vi "main.vi"() -> ()   [LabVIEW 2014]
uses:
  type definitions/control camera properties.ctl
  type definitions/state machine enum.ctl
  <vilib>/userdefined/High Color/IMAQdx.ctl
  <vilib>/vision/driver/NI_Vision_Acquisition_Software.lvlib
panel:
  out "Vertical Pixel Size":dbl
  out "Horizontal Pixel Size":dbl
  out "path":path
  out "bolean intcal":bool
  out "XY Graph":cluster{i32[], u32[]}(graph)
  out "Path to save:":path caption="Path"
  in  "Control Camera Properties":T1={"Packet Size"=1500, "Pixel Format"=17825797, "Gain in dB"=1.0, "Exposure Time in µs"=1500, "Stream Bytes per Second"=50000017} {"Stream Bytes per Second" min=1000000 max=124000000 step=100000 format="%.1p"; "Exposure Time in µs" min=21 max=153391689 format="%#.0f"; "Gain in dB" min=0.0 max=26.0 format="%#_2g"; "Pixel Format" items=["Mono 12 Packed"=17563654, "Mono 12"=17825797]}
  out "Image Pixels (U16)":u16[][](graph)
  in  "Stop Grab 2":bool
  in  "Calibration Button":bool
  out "Camera":T2
  in  "select camera":bool
  in  "Stop Button":bool
  in  "Snap Button":bool
  in  "Grab Button":bool
  in  "Save As Button":bool
  in  "Save Button":bool
  # "Camera Image:"
  # "Spectrum:"
  # "Bytes"
  # "px"
  # "px"
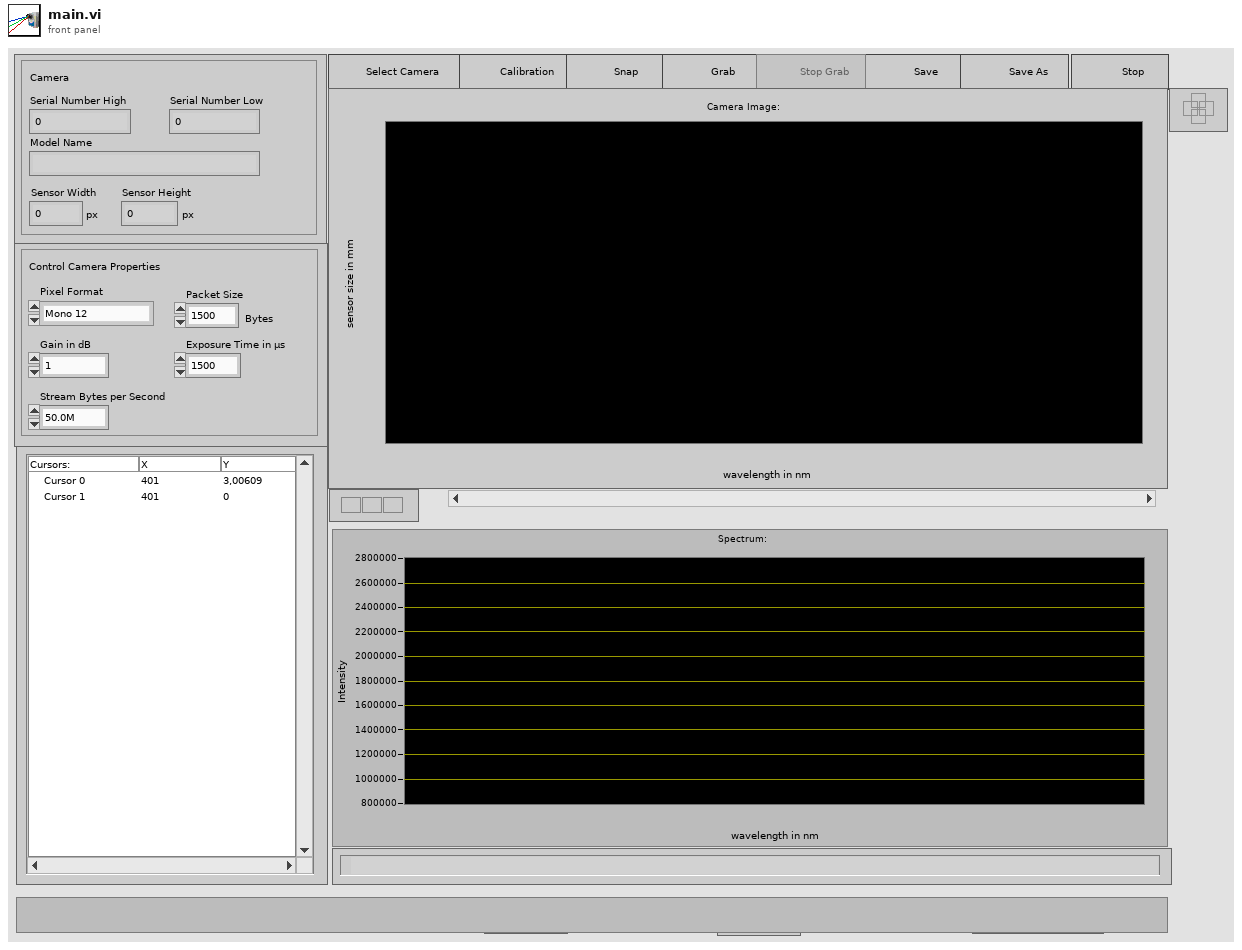
[diagram p1: front panel]
types:
  T1 = typedef "control camera properties.ctl" = cluster{"Packet Size":u32, "Pixel Format":u32, "Gain in dB":dbl, "Exposure Time in µs":u32, "Stream Bytes per Second":u32}
  T2 = cluster{"Serial Number High":u32, "Model Name":string, "Sensor Width":u32, "Sensor Height":u32, "Serial Number Low":u32}
  T3 = typedef "IMAQdx.ctl" = refnum<k21>
  T4 = typedef "state machine enum.ctl" = enum16{"start", "select camera", "read calibration data", "control camera properties", "calibration", "wait", "snap", "save", "save as", "grab", "error", "stop"}
  T5 = enum8{"Enabled", "Disabled", "Disabled and Grayed Out"}
  T6 = cluster{"boolean In":bool, "path In":path, "XScale.NameLbl.Text":string, "XScale.Multiplier":dbl, "XScale.Offset":dbl, "XScale.Minimum":dbl, "XScale.Maximum":dbl, "YScale.NameLbl.Text":string, "YScale.Multiplier":dbl, "YScale.Minimum":dbl, "YScale.Maximum":dbl}
  T7 = typedef "Image Type" = u32
  T8 = typedef "IMAQ Image.ctl" = refnum<image>
  T9 = cluster{"Value":bool, "Value":path, "XScale.NameLbl.Text":string, "XScale.Multiplier":dbl, "XScale.Offset":dbl, "XScale.Minimum":dbl, "XScale.Maximum":dbl, "YScale.NameLbl.Text":string, "YScale.Multiplier":dbl, "YScale.Minimum":dbl, "YScale.Maximum":dbl}
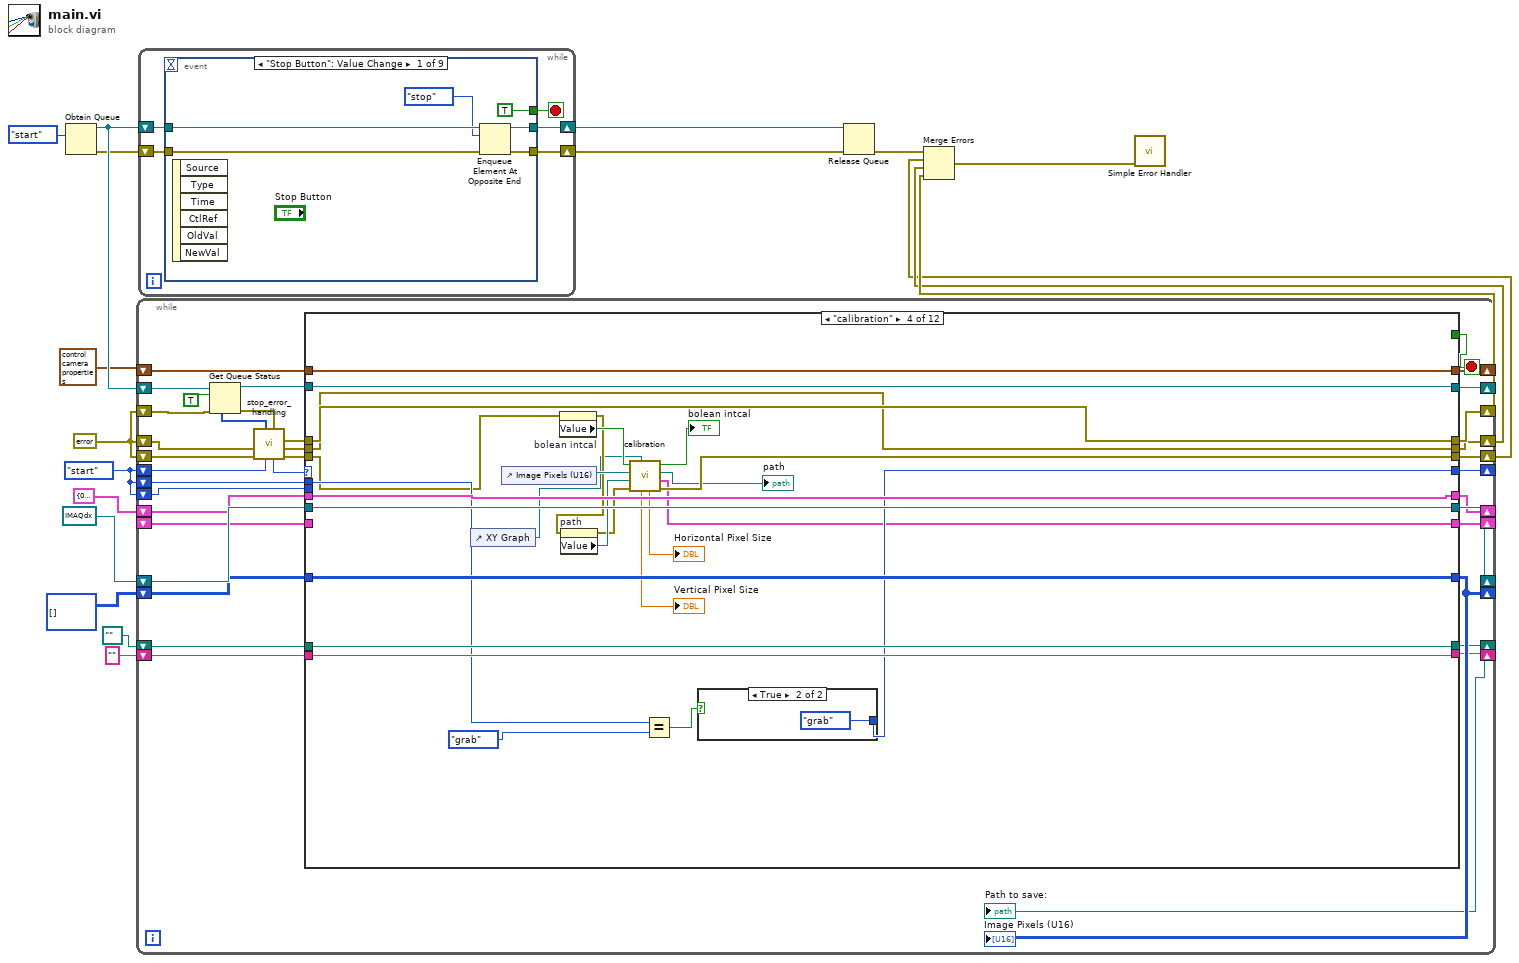
[diagram p0: block diagram]
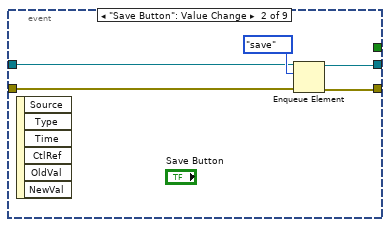
[diagram p2: hidden frame]
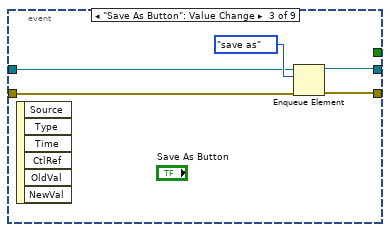
[diagram p3: hidden frame]
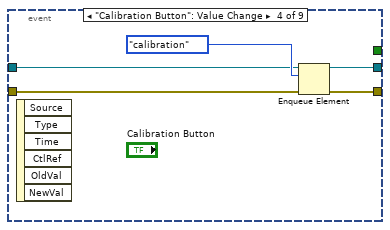
[diagram p4: hidden frame]
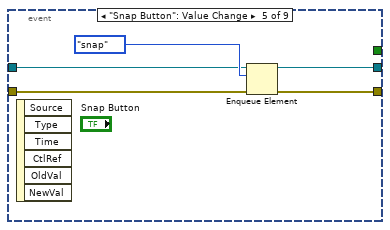
[diagram p5: hidden frame]
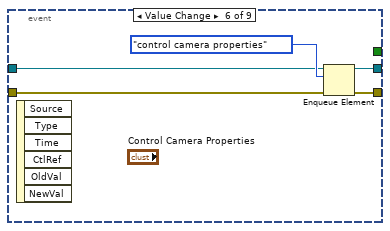
[diagram p6: hidden frame]
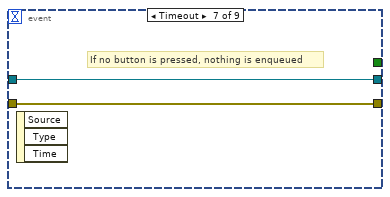
[diagram p7: hidden frame]
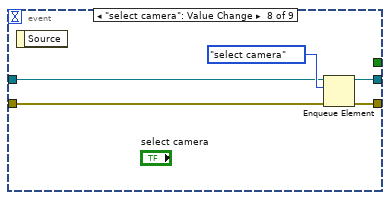
[diagram p8: hidden frame]
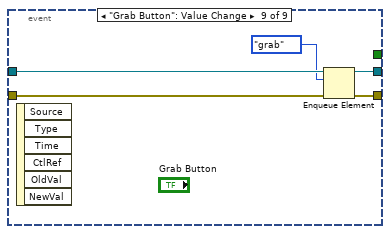
[diagram p9: hidden frame]
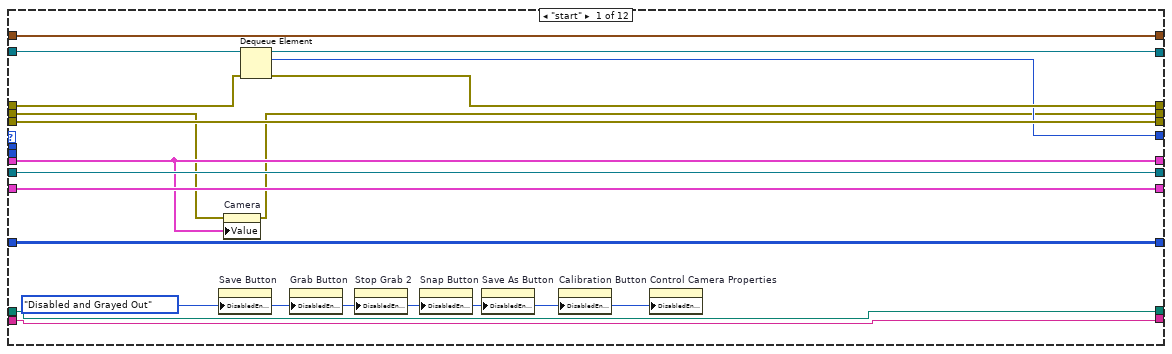
[diagram p10: hidden frame]
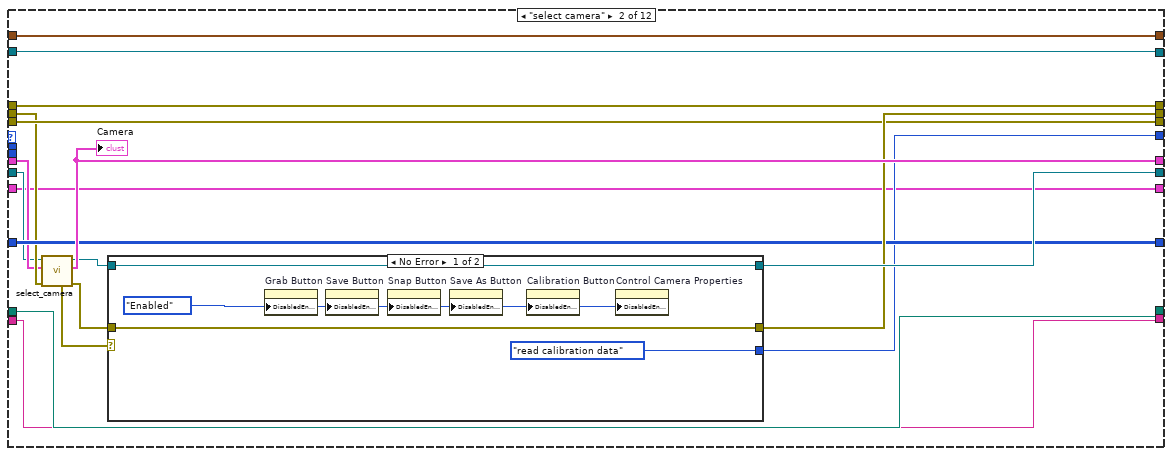
[diagram p11: hidden frame]
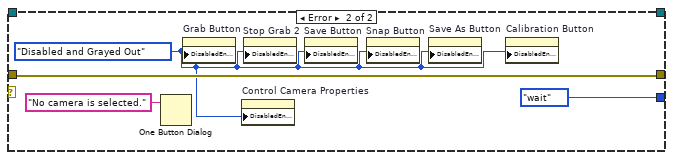
[diagram p12: hidden frame]
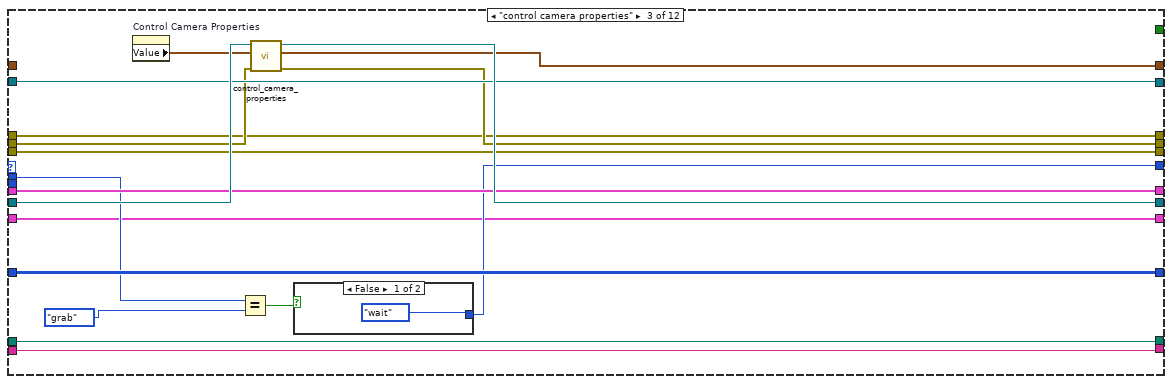
[diagram p13: hidden frame]
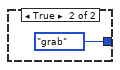
[diagram p14: hidden frame]
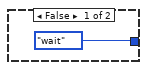
[diagram p15: hidden frame]
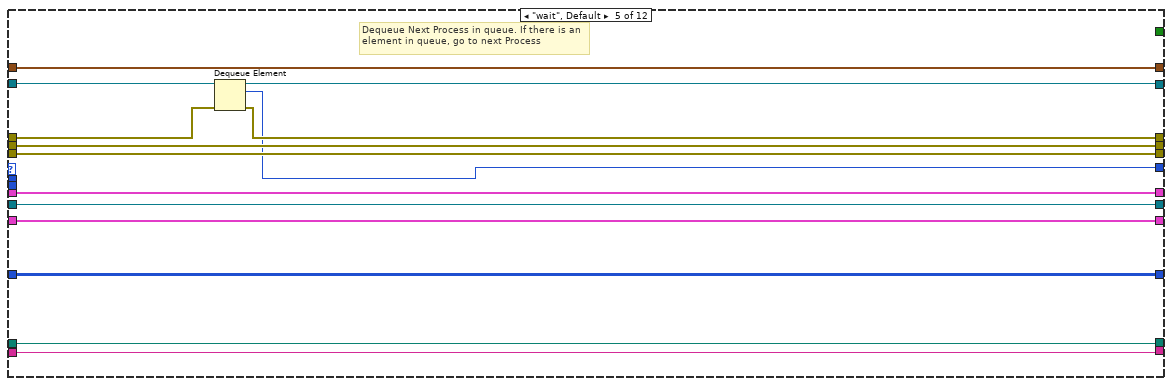
[diagram p16: hidden frame]
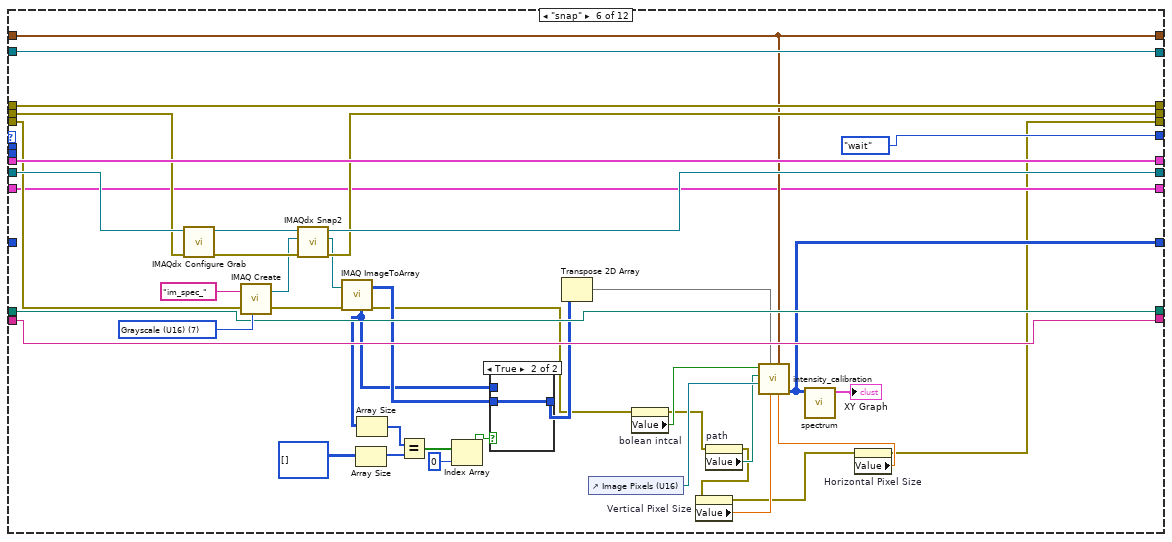
[diagram p17: hidden frame]
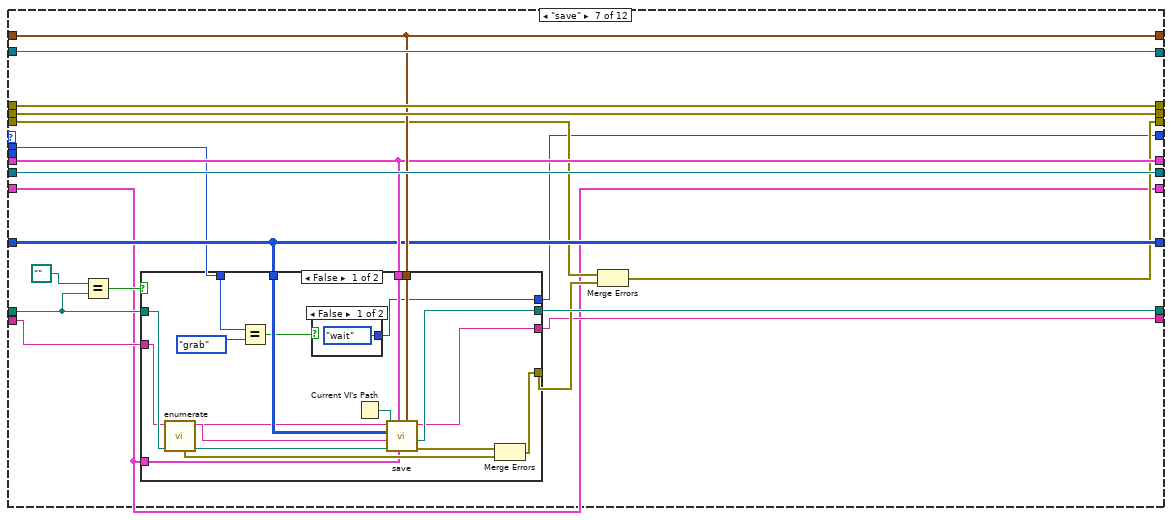
[diagram p19: hidden frame]
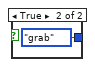
[diagram p20: hidden frame]
diagram:
  w9 = errorcluster {"status"=FALSE, "code"=0, "source"=""} ("error out")
  w1 = state_machine_enum."start" ("Zustände")
  n1 = Obtain Queue(element data type=state_machine_enum."start" ("Zustände")) -> (queue out=w18:refnum<queue>, error out=w12:errorcluster)  [unwired: 4 in, 1 out]
  n2 = while {
    shift-right: [w42] -> _
    shift-left: T1 {"Packet Size"=1500, "Pixel Format"=17825797, "Gain in dB"=1.0, "Exposure Time in µs"=1500, "Stream Bytes per Second"=50000017} ("Control Camera Properties 3") -> [w53]
    shift-right: [w50] -> w6
    shift-left: w9 -> [w39]
    shift-right: [w52] -> _
    shift-left: T3 refnum ("Session Out 2") -> [w51]
    shift-right: [w49] -> _
    shift-left: w18 -> [w47]
    shift-right: [w44] -> _
    shift-left: T2 {"Serial Number High"=0, "Model Name"="no device", "Sensor Width"=0, "Sensor Height"=0, "Serial Number Low"=0} ("Camera 2") -> [w43]
    shift-right: [w29] -> w5
    shift-left: w9 -> [w35]
    shift-right: [w38] -> w4
    shift-left: w9 -> [w31]
    shift-right: [w41] -> _
    shift-left: u16[][] [] -> [w40]
    shift-right: [w28] -> _
    shift-left: path "" ("appended path") -> [w26]
    shift-right: [w27] -> _
    shift-left: "" ("File Name Output") -> [w25]
    shift-right: [w22] -> _
    shift-left: w1 -> [w24]
    shift-left: w1 -> [w23]
    shift-left: w1 -> [w21]
    shift-right: [w20] -> _
    shift-left: _ -> [w19]
    stop <- w48 stop-if-true
    n3 = Get Queue Status(queue=w47, return elements? (F)=TRUE, error in (no error)=w39) -> (queue out=w46:refnum<queue>, error out=w37:errorcluster, elements=w36:T4[])  [unwired: 5 out]
    n4 = call "stop_error_handling.vi"("queue error in"=w37, "state in"=w24, "elements in queue"=w36, "image error in"=w31, "camera error in"=w35) -> ("image error out"=w32:errorcluster, "camera error out"=w33:errorcluster, "queue error out"=w34:errorcluster, "state out"=w30:T4)  [unwired: 3 in]
    n5 = case shown="\"calibration\"" w30 {
      tunnel: [w61 w87 w109 w141 w153 w170 w216 w250 w290 T1 {"Packet Size"=1500, "Pixel Format"=17563654, "Gain in dB"=1.0, "Exposure Time in µs"=1500, "Stream Bytes per Second"=50000017} ("Control Camera Properties 2") w419 w490] -> w42
      tunnel: w53 -> [w61 w87 _ w141 w153 w170 w216 w250 w290 _ w419 w490]
      tunnel: w34 -> [w68 w78 w105 w138 w156 w190 w218 w260 w307 w384 w414 w492]
      tunnel: [_ _ _ _ _ _ _ _ _ TRUE _ _] -> w48
      tunnel: [w69 w86 w112 w135 w152 w193 w220 w256 w314 w387 w415 w483] -> w52
      tunnel: w51 -> [w69 w74 w113 w135 w152 w197 w220 w256 w315 w390 w422 w483]
      tunnel: [w66 w78 w105 w138 w154 w190 w218 w260 w297 w384 w405 w492] -> w50
      tunnel: [w65 w85 w111 w139 w155 w191 w219 w258 w299 w392 w418 w491] -> w49
      tunnel: w46 -> [w67 w85 w111 w139 w157 w191 w219 w258 w309 w392 w418 w491]
      tunnel: [w56 w82 w110 w140 w151 w192 w215 w257 w313 w388 w417 w489] -> w44
      tunnel: w43 -> [w56 w75 w110 w140 w151 w192 w215 w257 w313 _ w417 w489]
      tunnel: w33 -> [w55 w76 w108 w137 w150 w189 w217 w259 w312 w386 w413 w493]
      tunnel: [w54 w80 w107 w137 w150 w188 w217 w259 w310 w385 w404 w493] -> w29
      tunnel: w32 -> [w64 w79 w106 w120 w149 w187 w210 w251 w311 w380 w412 w496]
      tunnel: [w64 w79 w106 w131 w149 w158 w209 w253 w306 w380 w403 w494] -> w38
      tunnel: [w62 w77 w103 w136 w148 w169 w214 w265 w308 _ w401 w488] -> w41
      tunnel: w40 -> [w62 w77 w103 w136 w148 _ w214 w264 _ _ w421 w488]
      tunnel: [w60 w73 w102 w134 w147 w184 w213 w255 w302 w382 w400 w487] -> w28
      tunnel: [w59 w72 w101 w133 w146 w183 w203 w254 w301 w381 w399 w486] -> w27
      tunnel: w26 -> [w60 w73 w102 w134 w147 w184 w207 _ w302 w382 w400 w487]
      tunnel: w25 -> [w59 w72 w101 w133 w146 w183 w212 _ w301 w381 w399 w486]
      tunnel: w23 -> [_ _ w98 w128 _ _ w205 w245 _ _ _ _]
      tunnel: [w58 w71 w97 w127 w145 state_machine_enum."wait" ("Zustände") w204 w246 w293 state_machine_enum."stop" ("Zustände") w398 state_machine_enum."control camera properties" ("Zustände")] -> w22
      tunnel: w21 -> [_ _ _ _ _ _ _ w247 _ _ _ _]
      tunnel: [w57 w70 w96 w124 w144 w167 w202 w244 w289 w378 w397 w498] -> w20
      tunnel: w19 -> [w57 w70 w96 _ w144 w167 w202 w244 w289 w378 w397 _]
      frame "start" {
        w63 = T5."Disabled and Grayed Out" ("Disabled")
        n6 = property on="Save Button" class="Bool"("DisabledEnum"=w63) -> ()  [unwired: 2 in, 2 out]
        n7 = property on="Camera" class="Clust (strict)"(error in=w55, "Value"=w56) -> (error out=w54:errorcluster)  [unwired: 1 in, 1 out]
        n8 = Dequeue Element(queue=w67, error in (no error)=w68) -> (queue out=w65:refnum<queue>, element=w58:T4, error out=w66:errorcluster)  [unwired: 1 in, 1 out]
        n9 = property on="Grab Button" class="Bool"("DisabledEnum"=w63) -> ()  [unwired: 2 in, 2 out]
        n10 = property on="Stop Grab 2" class="Bool"("DisabledEnum"=w63) -> ()  [unwired: 2 in, 2 out]
        n11 = property on="Snap Button" class="Bool"("DisabledEnum"=w63) -> ()  [unwired: 2 in, 2 out]
        n12 = property on="Save As Button" class="Bool"("DisabledEnum"=w63) -> ()  [unwired: 2 in, 2 out]
        n13 = property on="Calibration Button" class="Bool"("DisabledEnum"=w63) -> ()  [unwired: 2 in, 2 out]
        n14 = property on="Control Camera Properties" class="Clust (strict)"("DisabledEnum"=w63) -> ()  [unwired: 2 in, 2 out]
      }
      frame "select camera" {
        n15 = call "select_camera.vi"("Camera Error In"=w76, "Chosen Camera:"=w75, "Camera Session In"=w74) -> ("Camera Error Out"=w84:errorcluster, "Chosen Camera:"=w82:T2, "Camera Session Out"=w81:T3, "Session error"=w83:errorcluster)  [unwired: 5 in]
        "Camera" <- w82
        n16 = case shown="No Error" w83 {
          tunnel: w81 -> [w90 _]
          tunnel: w84 -> [w91 w93]
          tunnel: [w90 _] -> w86
          tunnel: [w91 w93] -> w80
          tunnel: [state_machine_enum."read calibration data" ("Zustände") state_machine_enum."wait" ("Zustände")] -> w71
          frame No Error {
            w88 = T5."Enabled" ("Disabled")
            n17 = property on="Grab Button" class="Bool"("DisabledEnum"=w88) -> ()  [unwired: 2 in, 2 out]
            n18 = property on="Save Button" class="Bool"("DisabledEnum"=w88) -> ()  [unwired: 2 in, 2 out]
            n19 = property on="Snap Button" class="Bool"("DisabledEnum"=w88) -> ()  [unwired: 2 in, 2 out]
            n20 = property on="Save As Button" class="Bool"("DisabledEnum"=w88) -> ()  [unwired: 2 in, 2 out]
            n21 = property on="Calibration Button" class="Bool"("DisabledEnum"=w88) -> ()  [unwired: 2 in, 2 out]
            n22 = property on="Control Camera Properties" class="Clust (strict)"("DisabledEnum"=w88) -> ()  [unwired: 2 in, 2 out]
          }
          frame Error {
            w92 = T5."Disabled and Grayed Out" ("Disabled")
            n23 = One Button Dialog(message="No camera is selected.") -> ()  [unwired: 1 in, 1 out]
            n24 = property on="Grab Button" class="Bool"("DisabledEnum"=w92) -> ()  [unwired: 2 in, 2 out]
            n25 = property on="Control Camera Properties" class="Clust (strict)"("DisabledEnum"=w92) -> ()  [unwired: 2 in, 2 out]
            n26 = property on="Stop Grab 2" class="Bool"("DisabledEnum"=w92) -> ()  [unwired: 2 in, 2 out]
            n27 = property on="Save Button" class="Bool"("DisabledEnum"=w92) -> ()  [unwired: 2 in, 2 out]
            n28 = property on="Snap Button" class="Bool"("DisabledEnum"=w92) -> ()  [unwired: 2 in, 2 out]
            n29 = property on="Save As Button" class="Bool"("DisabledEnum"=w92) -> ()  [unwired: 2 in, 2 out]
            n30 = property on="Calibration Button" class="Bool"("DisabledEnum"=w92) -> ()  [unwired: 2 in, 2 out]
          }
        }
      }
      frame "control camera properties" {
        n31 = property on="Control Camera Properties" class="Clust (strict)"() -> ("Value"=w104:T1)  [unwired: 2 in, 2 out]
        n32 = Equal?(x=w98, y=state_machine_enum."grab" ("Zustände")) -> (x = y?=w99:bool)
        n33 = call "control_camera_properties.vi"("error in (no error)"=w108, "Control Camera Properties"=w104, "IMAQdx Session"=w113) -> ("error out 2"=w107:errorcluster, "output cluster"=w109:T1, "Session Out 2"=w112:T3)  [unwired: 6 in]
        n34 = case shown="False" w99 {
          tunnel: [state_machine_enum."wait" ("Zustände") state_machine_enum."grab" ("Zustände")] -> w97
          frame False {
          }
          frame True {
          }
        }
      }
      frame "calibration" {
        n35 = control-ref of="XY Graph"() -> (w116:refnum<vi>)
        n36 = control-ref of="Image Pixels (U16)"() -> (w132:refnum<vi>)
        n37 = property on="bolean intcal" class="Bool (strict)"(error in=w120) -> (error out=w121:errorcluster, "Value"=w123:bool)  [unwired: 1 in, 1 out]
        n38 = property on="path" class="Path"(error in=w121) -> (error out=w119:errorcluster, "Value"=w122:path)  [unwired: 1 in, 1 out]
        n39 = call "calibration.vi"("xy graph reference"=w116, "graph error in"=w119, "path In"=w122, "reference"=w132, "intensity cal. boolean In"=w123) -> ("graph error out"=w131:errorcluster, "calibration info out"=w124:T6, "path out"=→"path":path, "boolean intcal out"=→"bolean intcal":bool, "Horizontal Pixel Size"=→"Horizontal Pixel Size":dbl, "Vertical Pixel Size"=→"Vertical Pixel Size":dbl)  [unwired: 1 in]
        n40 = Equal?(x=w128, y=state_machine_enum."grab" ("Zustände")) -> (x = y?=w129:bool)
        n41 = case shown="True" w129 {
          tunnel: [state_machine_enum."wait" ("Zustände") state_machine_enum."grab" ("Zustände")] -> w127
          frame False {
          }
          frame True {
          }
        }
      }
      frame "wait", Default {
        # "Dequeue Next Process in queue. If there is an element in queue, go to next Process"
        n42 = Dequeue Element(queue=w157, error in (no error)=w156) -> (queue out=w155:refnum<queue>, element=w145:T4, error out=w154:errorcluster)  [unwired: 1 in, 1 out]
      }
      frame "snap" {
        w199 = T7 7 items=["Grayscale (U8)", "Grayscale (I16)", "Grayscale (SGL)", "Complex (CSG)", "RGB (U32)", "HSL (U32)", "RGB (U64)", "Grayscale (U16)"] ("Image Type")
        n43 = call <vilib>:"IMAQdx Configure Grab.vi"("error in"=w189, "Session In"=w197) -> ("error out"=w196:errorcluster, "Session Out"=w195:T3)  [unwired: 8 in]
        n44 = call "IMAQ Create"("Image Name"="im_spec_", "Image Type"=w199, "error in (no error)"=w187) -> ("New Image"=w194:T8, "error out"=w185:errorcluster)  [unwired: 2 in]
        n45 = call <vilib>:"IMAQdx Snap2.vi"("error in"=w196, "Image In"=w194, "Session In"=w195) -> ("error out"=w188:errorcluster, "Image Out"=w186:T8, "Session Out"=w193:T3)  [unwired: 6 in]
        n46 = call "IMAQ ImageToArray"("error in (no error)"=w185, "Image"=w186) -> ("Image Pixels (U16)"=w174:u16[][], "error out"=w162:errorcluster, "Image Pixels (I16)"=w176:i16[][])  [unwired: 2 in, 2 out]
        n47 = Array Size(array=u16[][] []) -> (size(s)=w180:i32[])
        n48 = Array Size(array=w174) -> (size(s)=w182:i32[])
        n49 = Equal?(x=w182, y=w180) -> (x = y?=w179:bool[])
        n50 = Index Array(array=w179, index=0) -> (element=w177:bool)
        n51 = case shown="True" w177 {
          tunnel: w176 -> [_ w201]
          tunnel: [w200 w201] -> w175
          tunnel: w174 -> [w200 _]
          frame False {
          }
          frame True {
          }
        }
        n52 = Transpose 2D Array(2D array=w175) -> (transposed array=w171:u16[][])
        n53 = control-ref of="Image Pixels (U16)"() -> (w168:refnum<vi>)
        n54 = property on="bolean intcal" class="Bool (strict)"(error in=w162) -> (error out=w161:errorcluster, "Value"=w166:bool)  [unwired: 1 in, 1 out]
        n55 = property on="path" class="Path"(error in=w161) -> (error out=w160:errorcluster, "Value"=w165:path)  [unwired: 1 in, 1 out]
        n56 = property on="Vertical Pixel Size" class="DigNum (strict)"(error in=w160) -> (error out=w159:errorcluster, "Value"=w164:dbl)  [unwired: 1 in, 1 out]
        n57 = property on="Horizontal Pixel Size" class="DigNum (strict)"(error in=w159) -> (error out=w158:errorcluster, "Value"=w163:dbl)  [unwired: 1 in, 1 out]
        n58 = call "intensity_calibration.vi"("Horizontal Pixel Size 2"=w163, "Control Camera Properties"=w170, "Vertical Pixel Size 2"=w164, "array in"=w171, "reference"=w168, "appended path"=w165, "Boolean"=w166) -> ("array out"=w169:u16[][])  [unwired: 4 in]
        n59 = call "spectrum.vi"("Array"=w169) -> ("XY Graph"=→"XY Graph":cluster{i32[], u32[]})  [unwired: 10 in]
      }
      frame "save" {
        n60 = Equal?(x=path "" ("appended path"), y=w207) -> (x = y?=w206:bool)
        n61 = case shown="False" w206 {
          tunnel: w216 -> [w237 _]
          tunnel: w215 -> [w236 _]
          tunnel: w214 -> [w235 _]
          tunnel: w207 -> [w234 w243]
          tunnel: [w233 w243] -> w213
          tunnel: w212 -> [w227 _]
          tunnel: [w232 errorcluster {"status"=FALSE, "code"=0, "source"=""} ("error out")] -> w211
          tunnel: w205 -> [w223 _]
          tunnel: [w222 state_machine_enum."save as" ("Zustände")] -> w204
          tunnel: [w227 "" ("File Name Output")] -> w203
          tunnel: w202 -> [w221 _]
          frame False {
            n62 = call "enumerate.vi"("Path In"=w234, "Name Time Date In"=w227) -> ("Path Out"=w231:path, "Complete File Name Out"=w230:string, "path error out"=w229:errorcluster)  [unwired: 7 in]
            n63 = Equal?(x=w223, y=state_machine_enum."grab" ("Zustände")) -> (x = y?=w225:bool)
            n64 = case shown="False" w225 {
              tunnel: [state_machine_enum."wait" ("Zustände") state_machine_enum."grab" ("Zustände")] -> w222
              frame False {
              }
              frame True {
              }
            }
            n65 = Current VI's Path() -> (path=w226:path)
            n66 = call "save.vi"("Control Camera Properties 3"=w237, "calibration info"=w221, "Camera"=w236, "Path"=w231, "Complete File Name In"=w230, "Array"=w235, "path"=w226) -> ("saving error out"=w228:errorcluster, "Path out"=w233:path)  [unwired: 3 in]
            n67 = Merge Errors(w228, w229) -> (w232:errorcluster)
          }
          frame True {
          }
        }
        n68 = Merge Errors(w210, w211) -> (w209:errorcluster)
      }
      frame "save as" {
        n69 = Array Size(array=w264) -> (size(s)=w263:i32[])
        n70 = Index Array(array=w263) -> (element=w261:i32)  [unwired: 1 in]
        n71 = Equal To 0?(x=w261) -> (x = 0?=w262:bool)
        n72 = Equal?(x=state_machine_enum."save" ("Zustände"), y=w245) -> (x = y?=w248:bool)
        n73 = case shown="False" w262 {
          tunnel: w264 -> [w283 w287]
          tunnel: [w283 w287] -> w265
          tunnel: w250 -> [w285 _]
          tunnel: w257 -> [w284 _]
          tunnel: [w282 _] -> w255
          tunnel: [w281 _] -> w254
          tunnel: [w280 errorcluster {"status"=FALSE, "code"=0, "source"=""} ("error out")] -> w252
          tunnel: w244 -> [w278 _]
          frame False {
            n74 = Current VI's Path() -> (path=w279:path)
            n75 = call "save_as.vi"("calibration info"=w278, "Array"=w283, "Camera"=w284, "Control Camera Properties 3"=w285, "path"=w279) -> ("saving error out"=w280:errorcluster, "Name Time Date Out"=w281:string, "Path out"=w282:path)  [unwired: 4 in]
          }
          frame True {
            n76 = One Button Dialog(message="There is no image than can be saved. \nGrab or Snap to generate data before saving.") -> ()  [unwired: 1 in, 1 out]
          }
        }
        n77 = case shown="False" w248 {
          tunnel: w247 -> [_ w274]
          tunnel: [w266 w272] -> w246
          tunnel: w245 -> [w267 _]
          frame False {
            n78 = Equal?(x=w267, y=state_machine_enum."grab" ("Zustände")) -> (x = y?=w268:bool)
            n79 = case shown="False" w268 {
              tunnel: [state_machine_enum."wait" ("Zustände") state_machine_enum."grab" ("Zustände")] -> w266
              frame False {
              }
              frame True {
              }
            }
          }
          frame True {
            n80 = Equal?(x=state_machine_enum."grab" ("Zustände"), y=w274) -> (x = y?=w273:bool)
            n81 = case shown="False" w273 {
              tunnel: [state_machine_enum."wait" ("Zustände") state_machine_enum."grab" ("Zustände")] -> w272
              frame False {
              }
              frame True {
              }
            }
          }
        }
        n82 = Merge Errors(w251, w252) -> (w253:errorcluster)
      }
      frame "grab" {
        w317 = T7 7 items=["Grayscale (U8)", "Grayscale (I16)", "Grayscale (SGL)", "Complex (CSG)", "RGB (U32)", "HSL (U32)", "RGB (U64)", "Grayscale (U16)"] ("Image Type")
        n83 = call <vilib>:"IMAQdx Configure Grab.vi"("error in"=w312, "Session In"=w315) -> ("error out"=w304:errorcluster, "Session Out"=w316:T3)  [unwired: 8 in]
        n84 = property on="Stop Grab 2" class="Bool"("DisabledEnum"=T5."Enabled" ("Disabled")) -> ()  [unwired: 2 in, 2 out]
        n85 = call "IMAQ Create"("Image Name"="im_spec", "Image Type"=w317, "error in (no error)"=w311) -> ("New Image"=w303:T8, "error out"=w320:errorcluster)  [unwired: 2 in]
        n86 = while {
          shift-right: [w366] -> _
          shift-left: w303 -> [w368]
          shift-right: [w371] -> w318
          shift-left: w316 -> [w357]
          shift-right: [w325] -> w306
          shift-left: w320 -> [w367]
          shift-right: [w369] -> w319
          shift-left: w304 -> [w370]
          tunnel: w309 -> [w365]
          tunnel: [w338] -> w308
          tunnel: w307 -> [w362]
          tunnel: [w361] -> w298
          tunnel: [w345] -> w291
          tunnel: ["Stop Grab 2"] -> w296
          tunnel: w290 -> [_]
          tunnel: w290 -> [w337]
          stop <- w360 stop-if-true
          n87 = call <vilib>:"IMAQdx Grab2.vi"("error in"=w370, "Image In"=w368, "Session In"=w357) -> ("error out"=w369:errorcluster, "Image Out"=w366:T8, "Session Out"=w371:T3)  [unwired: 5 in, 1 out]
          n88 = Array Size(array=u16[][] []) -> (size(s)=w354:i32[])
          n89 = Get Queue Status(queue=w365, error in (no error)=w362) -> (queue out=w345:refnum<queue>, error out=w346:errorcluster, # elements in queue=w347:i32)  [unwired: 1 in, 5 out]
          n90 = call "IMAQ ImageToArray"("error in (no error)"=w367, "Image"=w366) -> ("Image Pixels (U16)"=w350:u16[][], "error out"=w332:errorcluster, "Image Pixels (I16)"=w348:i16[][])  [unwired: 2 in, 2 out]
          n91 = Array Size(array=w350) -> (size(s)=w356:i32[])
          n92 = Equal?(x=w356, y=w354) -> (x = y?=w353:bool[])
          n93 = control-ref of="Image Pixels (U16)"() -> (w334:refnum<vi>)
          n94 = Index Array(array=w353, index=0) -> (element=w351:bool)
          n95 = case shown="True" w351 {
            tunnel: [w372 w373] -> w349
            tunnel: w350 -> [w372 _]
            tunnel: w348 -> [_ w373]
            frame False {
            }
            frame True {
            }
          }
          n96 = Not Equal?(x=w347, y=0) -> (x != y?=w363:bool)
          n97 = Or(x=w363, y="Stop Grab 2") -> (x .or. y?=w359:bool)
          n98 = case shown="No Error" w346 {
            selector: w346 -> [w375 w377]
            tunnel: [w375 w377] -> w361
            tunnel: [FALSE TRUE] -> w358
            frame No Error {
            }
            frame Error {
            }
          }
          n99 = property on="bolean intcal" class="Bool (strict)"(error in=w332) -> (error out=w333:errorcluster, "Value"=w336:bool)  [unwired: 1 in, 1 out]
          n100 = property on="path" class="Path"(error in=w333) -> (error out=w329:errorcluster, "Value"=w335:path)  [unwired: 1 in, 1 out]
          n101 = Transpose 2D Array(2D array=w349) -> (transposed array=w339:u16[][])
          n102 = Wait (ms)(milliseconds to wait=u32 300) -> ()  [unwired: 1 out]
          n103 = property on="Vertical Pixel Size" class="DigNum (strict)"(error in=w329) -> (error out=w328:errorcluster, "Value"=w331:dbl)  [unwired: 1 in, 1 out]
          n104 = property on="Horizontal Pixel Size" class="DigNum (strict)"(error in=w328) -> (error out=w327:errorcluster, "Value"=w330:dbl)  [unwired: 1 in, 1 out]
          n105 = Or(x=w358, y=w359) -> (x .or. y?=w360:bool)
          n106 = property on="Property Node" class="IntGraph (strict)"(reference=w334, error in=w327) -> (error out=w326:errorcluster, "XScale.Multiplier"=w341:dbl, "XScale.Offset"=w340:dbl)  [unwired: 1 out]
          n107 = call "intensity_calibration.vi"("Horizontal Pixel Size 2"=w330, "Control Camera Properties"=w337, "Vertical Pixel Size 2"=w331, "array in"=w339, "reference"=w334, "appended path"=w335, "Boolean"=w336) -> ("array out"=w338:u16[][])  [unwired: 4 in]
          n108 = property on="Image Pixels (U16)" class="IntGraph (strict)"("Value"=w338) -> ()  [unwired: 2 in, 2 out]
          n109 = call "spectrum.vi"("Array"=w338) -> ("XY Graph"=w342:cluster{i32[], u32[]})  [unwired: 10 in]
          n110 = property on="XY Graph" class="XYGraph (strict)"(error in=w326, "Value"=w342, "XScale.Multiplier"=w341, "XScale.Offset"=w340) -> (error out=w325:errorcluster)  [unwired: 1 in, 1 out]
        }
        n111 = Equal?(x=w296, y=TRUE) -> (x = y?=w294:bool)
        n112 = call <vilib>:"IMAQdx Unconfigure Acquisition.vi"("error in"=w319, "Session In"=w318) -> ("error out"=w310:errorcluster, "Session Out"=w314:T3)  [unwired: 8 in]
        n113 = Dequeue Element(queue=w291, error in (no error)=w298) -> (queue out=w299:refnum<queue>, element=w292:T4, error out=w297:errorcluster)  [unwired: 1 in, 1 out]
        n114 = case shown="False" w294 {
          tunnel: [w322 state_machine_enum."wait" ("Zustände")] -> w293
          tunnel: w292 -> [w322 _]
          frame False {
            n115 = property on="Stop Grab 2" class="Bool"("DisabledEnum"=T5."Disabled and Grayed Out" ("Disabled")) -> ()  [unwired: 2 in, 2 out]
          }
          frame True {
            n116 = property on="Stop Grab 2" class="Bool"("DisabledEnum"=T5."Disabled and Grayed Out" ("Disabled")) -> ()  [unwired: 2 in, 2 out]
          }
        }
      }
      frame "stop" {
        w388 = T2 {"Serial Number High"=0, "Model Name"="no device", "Sensor Width"=0, "Sensor Height"=0, "Serial Number Low"=0} ("Camera 2")
        w387 = T3 refnum ("Session Out 2")
        n117 = Equal?(x=w390, y=w387) -> (x = y?=w391:bool)
        n118 = case shown="False" w391 {
          tunnel: w390 -> [w395 _]
          tunnel: [w394 w396] -> w385
          tunnel: w386 -> [w393 w396]
          frame False {
            n119 = call <vilib>:"IMAQdx Close Camera.vi"("error in"=w393, "Session In"=w395) -> ("error out"=w394:errorcluster)  [unwired: 9 in]
          }
          frame True {
          }
        }
        n120 = property on="Camera" class="Clust (strict)"("Value"=w388) -> ()  [unwired: 2 in, 2 out]
      }
      frame "error" {
        # "image error\nshow error, delete error, set array with image data to default, go to wait state"
        # "camera error\nshow error, close camera, delete error, and go back to start state"
        # "queue error\ndelete error, close camera and shut down program"
        n121 = case shown="Error" w414 {
          selector: w414 -> [w457 w472]
          tunnel: [w456 w471] -> w409
          tunnel: w413 -> [w461 w473]
          tunnel: [w461 w473] -> w410
          tunnel: [w457 w464] -> w411
          tunnel: w421 -> [w460 w470]
          tunnel: [w460 w470] -> w420
          tunnel: state_machine_enum."wait" ("Zustände") -> [w459 _]
          tunnel: [w459 state_machine_enum."stop" ("Zustände")] -> w424
          tunnel: w422 -> [w458 w466]
          tunnel: [w458 w462] -> w423
          tunnel: w412 -> [w456 w471]
          frame No Error {
          }
          frame Error {
            n122 = call <vilib>:"Clear Errors.vi"("error in (no error)"=w472) -> ("error out"=w465:errorcluster)  [unwired: 5 in, 1 out]
            n123 = Equal?(x=T3 refnum ("Session Out 2"), y=w466) -> (x = y?=w468:bool)
            n124 = case shown="False" w468 {
              tunnel: w466 -> [w478 w479]
              tunnel: [w477 w481] -> w464
              tunnel: w465 -> [w476 w481]
              tunnel: [TRUE ("stop? (T)") TRUE] -> w463
              tunnel: [T3 refnum ("Session Out 2") w479] -> w462
              frame False {
                n125 = call <vilib>:"IMAQdx Close Camera.vi"("error in"=w476, "Session In"=w478) -> ("error out"=w477:errorcluster)  [unwired: 9 in]
              }
              frame True {
              }
            }
            n126 = Stop(stop? (T)=w463) -> ()
          }
        }
        n127 = case shown="Error" w410 {
          selector: w410 -> [w442 w453]
          tunnel: [w440 w454] -> w406
          tunnel: w420 -> [w445 w455]
          tunnel: [w445 w455] -> w416
          tunnel: w409 -> [w440 w454]
          tunnel: w411 -> [w443 w452]
          tunnel: [w442 w448] -> w407
          tunnel: [w443 w452] -> w408
          tunnel: w424 -> [w444 _]
          tunnel: [w444 state_machine_enum."start" ("Zustände")] -> w402
          tunnel: w423 -> [w441 w447]
          tunnel: [w441 T3 refnum ("Session Out 2")] -> w415
          frame No Error {
          }
          frame Error {
            n128 = call <vilib>:"Simple Error Handler.vi"("error in (no error)"=w453) -> ("error out"=w450:errorcluster)  [unwired: 4 in, 4 out]
            n129 = call <vilib>:"IMAQdx Close Camera.vi"("error in"=w450, "Session In"=w447) -> ("error out"=w449:errorcluster)  [unwired: 9 in]
            n130 = call <vilib>:"Clear Errors.vi"("error in (no error)"=w449) -> ("error out"=w448:errorcluster)  [unwired: 5 in, 1 out]
          }
        }
        n131 = case shown="Error" w406 {
          selector: w406 -> [w431 w439]
          tunnel: [w431 w437] -> w403
          tunnel: w407 -> [w430 w435]
          tunnel: [w430 w435] -> w404
          tunnel: w408 -> [w429 w434]
          tunnel: [w429 w434] -> w405
          tunnel: w416 -> [w428 _]
          tunnel: [w428 u16[][] []] -> w401
          tunnel: w415 -> [w427 w433]
          tunnel: [w427 w433] -> _
          tunnel: w402 -> [w426 _]
          tunnel: [w426 state_machine_enum."wait" ("Zustände")] -> w398
          frame No Error {
          }
          frame Error {
            n132 = call <vilib>:"Simple Error Handler.vi"("error in (no error)"=w439) -> ("error out"=w438:errorcluster)  [unwired: 4 in, 4 out]
            n133 = call <vilib>:"Clear Errors.vi"("error in (no error)"=w438) -> ("error out"=w437:errorcluster)  [unwired: 5 in, 1 out]
          }
        }
      }
      frame "read calibration data" {
        n134 = property on="bolean intcal" class="Bool (strict)"(error in=w496) -> (error out=w495:errorcluster, "Value"=w482:bool)  [unwired: 1 in, 1 out]
        n135 = property on="path" class="Path"(error in=w495) -> (error out=w485:errorcluster, "Value"=w499:path)  [unwired: 1 in, 1 out]
        n136 = case shown="Error" w485 {
          selector: w485 -> [w510 w515]
          tunnel: [w510 w514] -> w484
          tunnel: w482 -> [_ w513]
          frame No Error {
          }
          frame Error {
            n137 = Equal?(x=w513, y=TRUE) -> (x = y?=w511:bool)
            n138 = case shown="True" w511 {
              frame False {
              }
              frame True {
                n139 = One Button Dialog(message="Invalid path for intensity calibration. \nTo change path, click on \"calibration\" \nand insert new path. ") -> ()  [unwired: 1 in, 1 out]
              }
            }
            n140 = call <vilib>:"Clear Errors.vi"("error in (no error)"=w515) -> ("error out"=w514:errorcluster)  [unwired: 5 in, 1 out]
          }
        }
        n141 = control-ref of="Image Pixels (U16)"() -> (w497:refnum<vi>)
        n142 = property on="Property Node" class="IntGraph (strict)"(reference=w497, error in=w484) -> (error out=w494:errorcluster, "XScale.NameLbl.Text"=w500:string, "XScale.Multiplier"=w501:dbl, "XScale.Offset"=w502:dbl, "XScale.Minimum"=w503:dbl, "XScale.Maximum"=w504:dbl, "YScale.NameLbl.Text"=w505:string, "YScale.Multiplier"=w506:dbl, "YScale.Minimum"=w507:dbl, "YScale.Maximum"=w508:dbl)  [unwired: 1 out]
        n143 = Bundle("Value"=w482, "Value"=w499, "XScale.NameLbl.Text"=w500, "XScale.Multiplier"=w501, "XScale.Offset"=w502, "XScale.Minimum"=w503, "XScale.Maximum"=w504, "YScale.NameLbl.Text"=w505, "YScale.Multiplier"=w506, "YScale.Minimum"=w507, "YScale.Maximum"=w508) -> (w498:T9)  [unwired: 1 in]
      }
    }
    "Image Pixels (U16)" <- w41
    "Path to save:" <- w28
  }
  n144 = while {
    shift-right: [w520] -> w17
    shift-left: w12 -> [w518]
    shift-right: [w519] -> w13
    shift-left: w18 -> [w521]
    stop <- w517 stop-if-true
    n145 = event shown="[0] \"Stop Button\": Value Change" {
      selector: _ -> [_ _ _ _ _ _ _ _ _]
      dyn-events: _ -> [_ _ _ _ _ _ _ _ _]
      timeout: _ -> [_ _ _ _ _ _ _ _ _]
      tunnel: w521 -> [w527 w531 w536 w541 w546 w551 w554 w558 w564]
      tunnel: [w524 w528 w533 w539 w544 w548 w553 w557 w562] -> w520
      tunnel: [TRUE _ _ _ _ _ _ _ _] -> w517
      tunnel: [w523 w529 w535 w538 w545 w550 w554 w556 w563] -> w519
      tunnel: w518 -> [w522 w530 w534 w540 w543 w549 w553 w555 w560]
      event "Stop Button": Value Change {
        n146 = event-data() -> ()  [unwired: 1 in, 6 out]
        n147 = Enqueue Element At Opposite End(queue=w527, element=state_machine_enum."stop" ("Zustände"), error in (no error)=w522) -> (queue out=w523:refnum<queue>, error out=w524:errorcluster)  [unwired: 1 in, 1 out]
      }
      event "Save Button": Value Change {
        n148 = event-data() -> ()  [unwired: 1 in, 6 out]
        n149 = Enqueue Element(queue=w531, element=state_machine_enum."save" ("Zustände"), error in (no error)=w530) -> (queue out=w529:refnum<queue>, error out=w528:errorcluster)  [unwired: 1 in, 1 out]
      }
      event "Save As Button": Value Change {
        n150 = event-data() -> ()  [unwired: 1 in, 6 out]
        n151 = Enqueue Element(queue=w536, element=state_machine_enum."save as" ("Zustände"), error in (no error)=w534) -> (queue out=w535:refnum<queue>, error out=w533:errorcluster)  [unwired: 1 in, 1 out]
      }
      event "Calibration Button": Value Change {
        n152 = event-data() -> ()  [unwired: 1 in, 6 out]
        n153 = Enqueue Element(queue=w541, element=state_machine_enum."calibration" ("Zustände"), error in (no error)=w540) -> (queue out=w538:refnum<queue>, error out=w539:errorcluster)  [unwired: 1 in, 1 out]
      }
      event "Snap Button": Value Change {
        n154 = event-data() -> ()  [unwired: 1 in, 6 out]
        n155 = Enqueue Element(queue=w546, element=state_machine_enum."snap" ("Zustände"), error in (no error)=w543) -> (queue out=w545:refnum<queue>, error out=w544:errorcluster)  [unwired: 1 in, 1 out]
      }
      event Value Change {
        n156 = event-data() -> ()  [unwired: 1 in, 6 out]
        n157 = Enqueue Element(queue=w551, element=state_machine_enum."control camera properties" ("Zustände"), error in (no error)=w549) -> (queue out=w550:refnum<queue>, error out=w548:errorcluster)  [unwired: 1 in, 1 out]
      }
      event Timeout {
        # "If no button is pressed, nothing is enqueued"
        n158 = event-data() -> ()  [unwired: 1 in, 3 out]
      }
      event "select camera": Value Change {
        n159 = event-data() -> ()  [unwired: 1 in, 1 out]
        n160 = Enqueue Element(queue=w558, element=state_machine_enum."select camera" ("Zustände"), error in (no error)=w555) -> (queue out=w556:refnum<queue>, error out=w557:errorcluster)  [unwired: 1 in, 1 out]
      }
      event "Grab Button": Value Change {
        n161 = event-data() -> ()  [unwired: 1 in, 6 out]
        n162 = Enqueue Element(queue=w564, element=state_machine_enum."grab" ("Zustände"), error in (no error)=w560) -> (queue out=w563:refnum<queue>, error out=w562:errorcluster)  [unwired: 1 in, 1 out]
      }
    }
  }
  n163 = Release Queue(queue=w13, error in (no error)=w17) -> (error out=w15:errorcluster)  [unwired: 1 in, 2 out]
  n164 = Merge Errors(w15, w4, w5, w6) -> (w14:errorcluster)
  n165 = call <vilib>:"Simple Error Handler.vi"("error in (no error)"=w14) -> ()  [unwired: 4 in, 5 out]
